vi "DCPower_RECONFIGURE_VoltageOrChannelname_AfterJSONfile_REFERENCE_byChannel.vi"(3 "error in":errorcluster, 4 "ColorPalette":T2=[16711686, 65351, 8978420, 14474240, 16139007, 16752640, 8958719, 16758973, 16777215, 46792, 11992992, 12961221, 16763690, 12600063, 16711835, 2953983, 40796, 13111296, 13352613, 9221011, 12964076, 12819897, 65442, 16776704, 14540253, 16740729, 10658047, 10813344, 16753521, 13413843, 8691115, 10339240, 14401205, 16746704, 7467519, 16775978, 13872558, 11387603, 13354405, 10420227, 13107364, 4060, 35208, 11817216, 7566080, 40796, 7539456, 2837073, 6372186, 7499083, 10648702, 16757152], 5 "VISAPowerInfoInputArray":T3[](array[typedef]), 6 "DCPowerInformationArrayOutput_byChannel_input":T1(array[cluster])) -> (0 "error out":errorcluster, 1 "VISAPowerInfoOutputArray":T3[](array[typedef]), 2 "DCPowerInformationArrayOutput_byChannel_output":T1(array[cluster]))   [LabVIEW 2019]
uses:
  Controls/PlotColorArray.ctl
  Controls/VISA_power_Control.ctl
panel:
  in  "Current Reset Value (A)":dbl
  out "Measured Voltage":dbl[](array[numeric])
  out "Measured Currents":dbl[](array[numeric])
  out "Configuration Echo":string
  out "Parameter Configuration Echo":string[][](array[string])
  in  "Channel Names":string[](array[string])
  in  "Change VISA Configurations":bool
  in  "Combination Scheme":u16(ring) items=["OFF", "SERIES", "PARALLEL"]
  in  "Which Channels to Parallelize":u16(ring) items=["I1+I2", "ALL", "I2+I3"]
  in  "Current Limit Channel 3":dbl
  in  "Current Limit Channel 2":dbl
  in  "Current Limit Channel 1":dbl
  in  "Voltage Channel 3":dbl
  in  "Voltage Channel 2":dbl
  in  "Voltage Channel 1":dbl
  in  "visa power channel select":u16(ring) items=["GPIB0::3::INSTR; channel names :channel1,channel2,channel3"]
  in  "Power On":bool
  in  "Change DC Power Channel Name":bool
  in  "Change DC Power Voltage":bool
  out "Current Measured (A)":dbl
  out "Voltage Measured (V)":dbl
  in  "Channel Name (str)":string
  in  "Voltage Level (V)":dbl
  out "Current Measured All (A)":dbl[][](array[numeric])
  out "Voltage Measured All (V)":dbl[][](array[numeric])
  out "Current Waveform Array":waveform(dbl)[](graph)
  out "Voltage Waveform Array":waveform(dbl)[](graph)
  in  "dc power channel select":u16(ring) items=["Slot_4_PXIe4139; channel number:  0; channel name: Red 5v", "Slot_5_PXIe4139; channel number:  0; channel name: Orange 3.3v_6780", "Slot_6_PXIe4139; channel number:  0; channel name: Yellow 1.8v", "PXIe4163; channel number:  0; channel name: Green 3.3v", "PXIe4163; channel number:  1; channel name: Blue 2.6v VATT"]
  in  "End Reconfig":bool
  # "Nothing to see behind here, surely"
  # "Change Parameters"
  # "MEASURED OUTPUTS (MAY NEED TO PRESS APPLY A FEW TIMES TO SEE ACTUAL OUTPUT)"
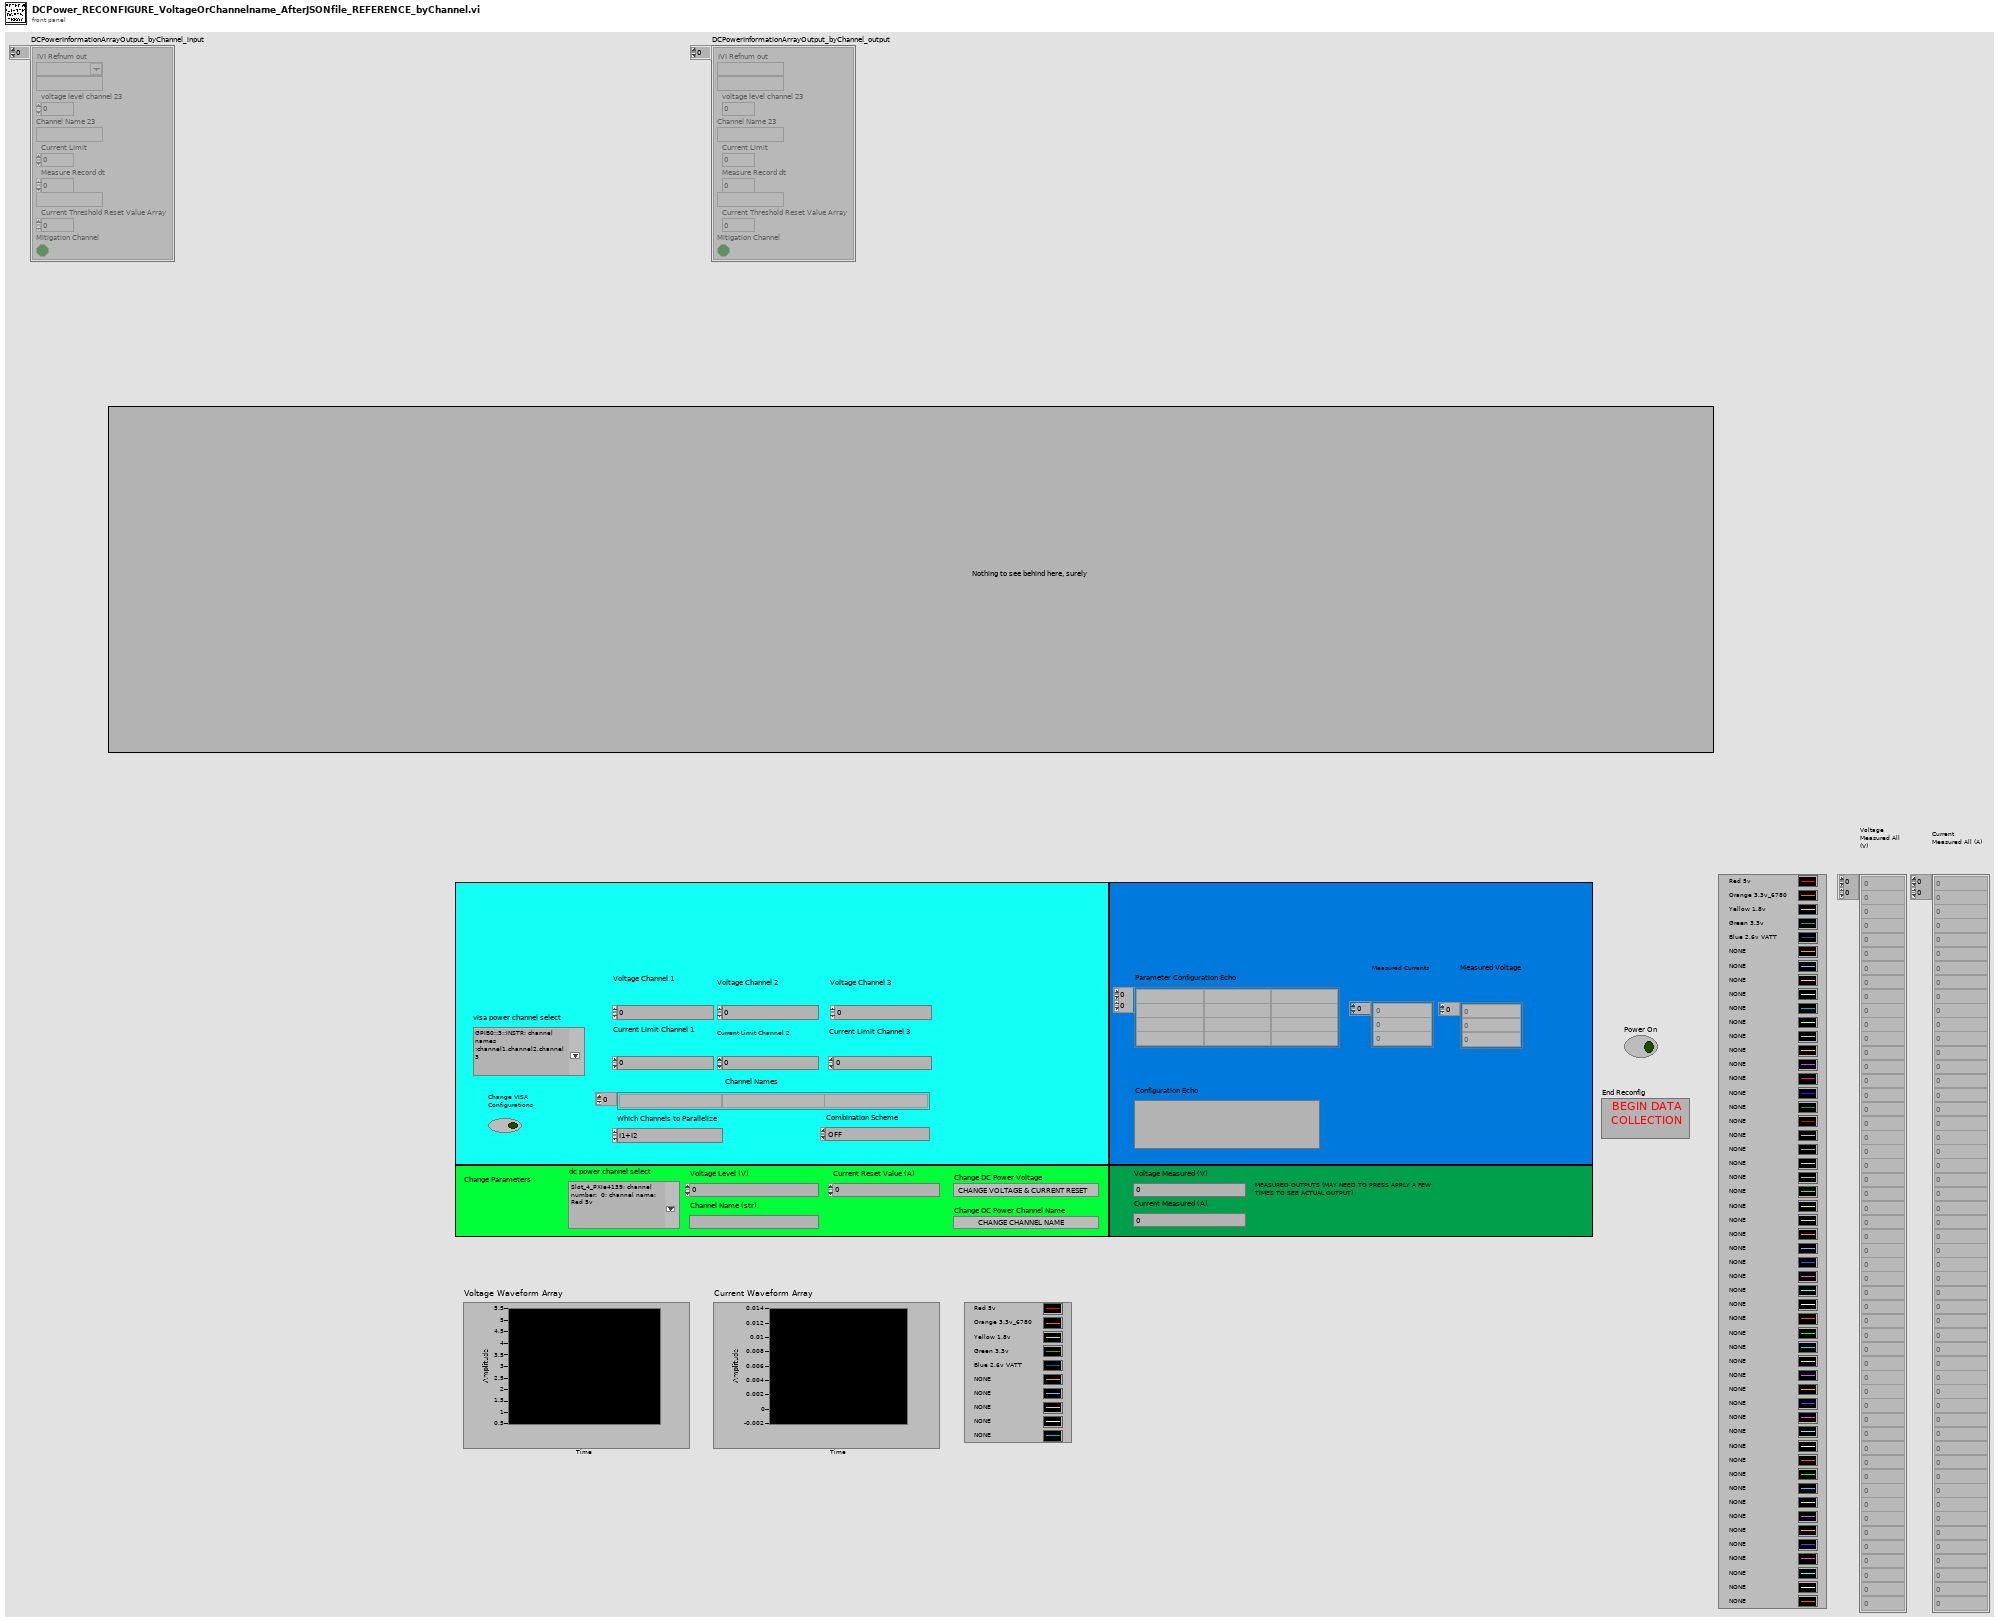
[diagram p1: front panel]
types:
  T1 = cluster{"IVI Refnum out":refnum<k15>, string, "voltage level channel 23":dbl, "Channel Name 23":string, "Current Limit":dbl, "Measure Record dt":dbl, string, "Current Threshold Reset Value Array":dbl, "Mitigation Channel":bool}[]
  T2 = typedef "PlotColorArray.ctl" = u32[]
  T3 = typedef "VISA_power_Control.ctl" = cluster{"VISA resource name":refnum<visa-resource-name>, "Active Channel List":string, "Active Channel Array":string[], "Input Array (Voltage,Current_Limit)":dbl[], "Input Array (Voltage,Current_Limit)":dbl[], "Channel Names":string[], "read buffer":string, "Channel Names Array":string[]}
  T4 = cluster{"IVI Refnum out":refnum<k15>, string, "voltage level channel 23":dbl, "Channel Name 23":string, "Current Limit":dbl, "Measure Record dt":dbl, string}[]
  T5 = typedef "LVStringsAndValuesArrayTypeDef_U16.ctl" = cluster{"String":string, "Value":u16}[]
  T6 = cluster{"VISA resource name":refnum<visa-resource-name>, "Active Channel List":string, "Active Channel Array":string[], "Input Array (Voltage,Current_Limit)":dbl[], "Input Array (Voltage,Current_Limit)":dbl[], "Channel Names":string[], "read buffer":string, "Channel Names":string[]}
  T7 = cluster{"IVI Refnum out":refnum<k15>, string, "voltage level channel 23":dbl, "Channel Name 23":string, "Current Limit":dbl, "Measure Record dt":dbl, string, "Current Threshold Reset Value Array":dbl, "Mitigation Channel":bool}
  T8 = cluster{"IVI Refnum out":refnum<k15>, string, "voltage level channel 23":dbl, "Channel Name (str)":string, "Current Limit":dbl, "Measure Record dt":dbl, string, "Current Threshold Reset Value Array":dbl, "Mitigation Channel":bool}
  T9 = cluster{"instrument handle out":refnum<k15>, string, "Voltage Level (V)":dbl, "Channel Name 23":string, "Current Limit":dbl, "Measure Record dt":dbl, string, "Current Reset Value (A)":dbl, "Mitigation Channel":bool}
  T10 = cluster{"IVI Refnum out":refnum<k15>, "String List":string, string[], dbl[], string[], dbl[], dbl[], string[], dbl[], bool[]}[]
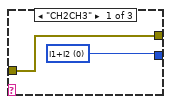
[diagram p4: hidden frame]
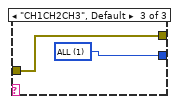
[diagram p5: hidden frame]
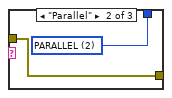
[diagram p6: hidden frame]
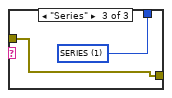
[diagram p7: hidden frame]
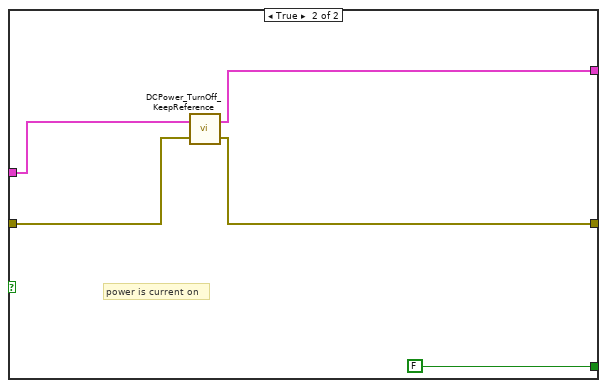
[diagram p9: hidden frame]
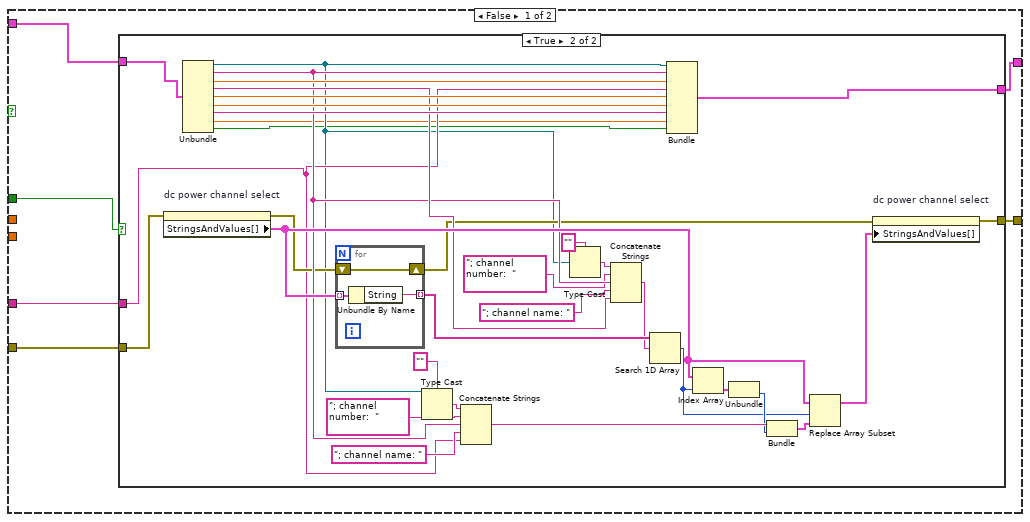
[diagram p10: hidden frame]
diagram:
  (unwired) T4 [] ("DCPowerInformation_byChannel_input")
  n1 = flat-sequence {
    tunnel: "DCPowerInformationArrayOutput_byChannel_input" -> [w16]
    tunnel: [w16] -> w12
    tunnel: [w15] -> w11
    tunnel: "error in" -> [w15]
    tunnel: [w13] -> w6
    tunnel: "VISAPowerInfoInputArray" -> [w13]
    tunnel: w12 -> [w34]
    tunnel: w11 -> [w47]
    tunnel: [w34] -> w10
    tunnel: [w17] -> w9
    tunnel: w6 -> [w28]
    tunnel: [w28] -> w5
    tunnel: w10 -> [w94]
    tunnel: w9 -> [w93]
    tunnel: [w92] -> w8
    tunnel: [w91] -> w1
    tunnel: w5 -> [w87]
    tunnel: [w86] -> w3
    frame #0 {
      n2 = local write "Power On"(FALSE ("Power On")) -> ()
    }
    frame #1 {
      n3 = Bundle("concatenated string"="pseudo", -1) -> (w46:cluster{"concatenated string":string, i32})  [unwired: 1 in]
      n4 = Build Array(w46) -> (w45:cluster{"concatenated string":string, i32}[])
      n5 = property on="dc power channel select" class="Ring (strict)"(error in=w47, "StringsAndValues[]"=w45) -> (error out=w48:errorcluster)  [unwired: 1 in, 1 out]
      n6 = property on="dc power channel select" class="Ring (strict)"(error in=w48) -> (error out=w49:errorcluster, "StringsAndValues[]"=w50:T5)  [unwired: 1 in, 1 out]
      n7 = for {
        tunnel: w34 -> [w76] mode=indexing
        shift-right: [w71] -> _
        shift-left: w50 -> [w73]
        shift-right: [w74] -> w42
        shift-left: w49 -> [w85]
        i -> [w75]
        n8 = Unbundle(w76) -> ("IVI Refnum out"=w84:refnum<k15>, w80:string, "Channel Name 23"=w78:string)  [unwired: 6 out]
        n9 = Type Cast(type="", x=w84) -> (*(type *) &x=w82:string)
        n10 = Concatenate Strings(w82, "; channel number:  " ("string"), w80, "; channel name: " ("string"), w78) -> (w77:string)
        n11 = Bundle(w77, w75) -> (w72:cluster{string, i32})  [unwired: 1 in]
        n12 = Build Array (concatenate)(w73, w72) -> (w71:cluster{"String":string, "Value":i32}[])
        n13 = property on="dc power channel select" class="Ring (strict)"(error in=w85, "StringsAndValues[]"=w71) -> (error out=w74:errorcluster)  [unwired: 1 in, 1 out]
      }
      n14 = property on="dc power channel select" class="Ring (strict)"(error in=w42) -> (error out=w41:errorcluster, "StringsAndValues[]"=w37:T5)  [unwired: 1 in, 1 out]
      n15 = for {
        tunnel: w37 -> [w70] mode=indexing
        shift-right: [w68] -> _
        shift-left: w41 -> [w68]
        tunnel: [w69] -> w39 mode=indexing
        n16 = Unbundle By Name(w70) -> ("Value"=w69:u16)
      }
      n17 = Search 1D Array(1D array=w39, element=u16 65535) -> (index of element=w40:i32)  [unwired: 1 in]
      n18 = Delete From Array(array=w37, index=w40) -> (array with subset deleted=w36:T5)  [unwired: 1 in, 1 out]
      n19 = property on="dc power channel select" class="Ring (strict)"(error in=w41, "StringsAndValues[]"=w36) -> (error out=w35:errorcluster)  [unwired: 1 in, 1 out]
      n20 = property on="dc power channel select" class="Ring (strict)" props=["StringsAndValues[]"](error in=w35) -> (error out=w29:errorcluster)  [unwired: 1 in, 2 out]
      n21 = Bundle("concatenated string"="pseudo", -1) -> (w31:cluster{"concatenated string":string, i32})  [unwired: 1 in]
      n22 = Build Array(w31) -> (w30:cluster{"concatenated string":string, i32}[])
      n23 = property on="visa power channel select" class="Ring (strict)"(error in=w29, "StringsAndValues[]"=w30) -> (error out=w27:errorcluster)  [unwired: 1 in, 1 out]
      n24 = property on="visa power channel select" class="Ring (strict)"(error in=w27) -> (error out=w26:errorcluster, "StringsAndValues[]"=w25:T5)  [unwired: 1 in, 1 out]
      n25 = for {
        shift-right: [w56] -> w24
        shift-left: w26 -> [w57]
        shift-right: [w55] -> _
        shift-left: w25 -> [w58]
        tunnel: w28 -> [w67] mode=indexing
        i -> [w60]
        n26 = Unbundle(w67) -> ("VISA resource name"=w66:refnum<visa-resource-name>, "Channel Names Array"=w54:string[])  [unwired: 6 out]
        n27 = call "StringArray2StringList.vi"("String Array"=w54) -> ("String List"=w62:string)
        n28 = Type Cast(type="", x=w66) -> (*(type *) &x=w64:string)
        n29 = Concatenate Strings(w64, "; channel names :" ("string"), w62) -> (w61:string)
        n30 = Bundle(w61, w60) -> (w59:cluster{string, i32})  [unwired: 1 in]
        n31 = Build Array (concatenate)(w58, w59) -> (w55:cluster{"String":string, "Value":i32}[])
        n32 = property on="visa power channel select" class="Ring (strict)"(error in=w57, "StringsAndValues[]"=w55) -> (error out=w56:errorcluster)  [unwired: 1 in, 1 out]
      }
      n33 = property on="visa power channel select" class="Ring (strict)"(error in=w24) -> (error out=w18:errorcluster, "StringsAndValues[]"=w20:T5)  [unwired: 1 in, 1 out]
      n34 = for {
        tunnel: w20 -> [w53] mode=indexing
        shift-right: [w51] -> _
        shift-left: w20 -> [w51]
        tunnel: [w52] -> w22 mode=indexing
        n35 = Unbundle By Name(w53) -> ("Value"=w52:u16)
      }
      n36 = Search 1D Array(1D array=w22, element=u16 65535) -> (index of element=w23:i32)  [unwired: 1 in]
      n37 = Delete From Array(array=w20, index=w23) -> (array with subset deleted=w19:T5)  [unwired: 1 in, 1 out]
      n38 = property on="visa power channel select" class="Ring (strict)"(error in=w18, "StringsAndValues[]"=w19) -> (error out=w17:errorcluster)  [unwired: 1 in, 1 out]
    }
    frame #2 {
      n39 = while {
        shift-right: [w95] -> w91
        shift-left: w94 -> [w138]
        shift-right: [w118] -> w92
        shift-left: w93 -> [w114]
        tunnel: "ColorPalette" -> [w136]
        shift-right: [w124] -> _
        shift-left: FALSE (".not. x?") -> [w102]
        shift-right: [w109] -> _
        shift-left: u16 0 -> [w106]
        shift-right: [w98] -> w86
        shift-left: w87 -> [w110]
        i -> [w105]
        stop <- w137 stop-if-true
        # "Need to add channel number cofiguration(position eventually)"
        n40 = property on="visa power channel select" class="Ring (strict)"(error in=w114) -> (error out=w113:errorcluster, "StringsAndValues[]"=w116:T5)  [unwired: 1 in, 1 out]
        n41 = Index Array(array=w116, index="visa power channel select") -> (element=w115:cluster{"String":string, "Value":u16})
        n42 = Unbundle(w115) -> ("Value"=w109:u16)  [unwired: 1 out]
        n43 = Not Equal?(x=w109, y=w106) -> (x != y?=w108:bool)
        n44 = Equal To 0?(x=w105) -> (x = 0?=w107:bool)
        n45 = Or(x=w108, y=w107) -> (x .or. y?=w104:bool)
        n46 = case shown="True" w104 {
          tunnel: w110 -> [_ w232]
          tunnel: w109 -> [_ w233]
          tunnel: [w197 w208] -> w112
          tunnel: w113 -> [w197 w211]
          frame False {
          }
          frame True {
            n47 = Index Array(array=w232, index=w233) -> (element=w231:T3)
            n48 = Unbundle(w231) -> ("Input Array (Voltage,Current_Limit)"=w221:dbl[], "Input Array (Voltage,Current_Limit)"=w220:dbl[], "Channel Names"=w207:string[], "read buffer"=w206:string)  [unwired: 4 out]
            n49 = Index Array(array=w221, index=0) -> (element=w225:dbl)
            n50 = call <vilib>:"Space Constant.vi"() -> ("String"=w205:string)
            n51 = property on="Voltage Channel 1" class="DigNum (strict)"(error in=w211, "Value"=w225) -> (error out=w230:errorcluster)  [unwired: 1 in, 1 out]
            n52 = Index Array(array=w221, index=1) -> (element=w224:dbl)
            n53 = Match Pattern(string=w206, regular expression=w205) -> (before substring=w204:string, after substring=w201:string)  [unwired: 1 in, 2 out]
            n54 = property on="Voltage Channel 2" class="DigNum (strict)"(error in=w230, "Value"=w224) -> (error out=w229:errorcluster)  [unwired: 1 in, 1 out]
            n55 = Index Array(array=w221, index=2) -> (element=w223:dbl)
            n56 = property on="Voltage Channel 3" class="DigNum (strict)"(error in=w229, "Value"=w223) -> (error out=w228:errorcluster)  [unwired: 1 in, 1 out]
            n57 = Index Array(array=w220, index=0) -> (element=w222:dbl)
            n58 = property on="Current Limit Channel 1" class="DigNum (strict)"(error in=w228, "Value"=w222) -> (error out=w226:errorcluster)  [unwired: 1 in, 1 out]
            n59 = Index Array(array=w220, index=1) -> (element=w219:dbl)
            n60 = property on="Current Limit Channel 2" class="DigNum (strict)"(error in=w226, "Value"=w219) -> (error out=w227:errorcluster)  [unwired: 1 in, 1 out]
            n61 = Index Array(array=w220, index=2) -> (element=w218:dbl)
            n62 = property on="Current Limit Channel 3" class="DigNum (strict)"(error in=w227, "Value"=w218) -> (error out=w203:errorcluster)  [unwired: 1 in, 1 out]
            n63 = case shown="\"NONE\", Default" w204 {
              tunnel: w203 -> [w240 w242 w244]
              tunnel: [w241 w243 w245] -> w202
              tunnel: [w240 w242 w244] -> w199
              frame "NONE", Default {
                w241 = u16 0 items=["OFF", "SERIES", "PARALLEL"] ("Combination Scheme")
              }
              frame "Parallel" {
                w243 = u16 2 items=["OFF", "SERIES", "PARALLEL"] ("Combination Scheme")
              }
              frame "Series" {
                w245 = u16 1 items=["OFF", "SERIES", "PARALLEL"] ("Combination Scheme")
              }
            }
            n64 = case shown="\"CH1CH2\"" w201 {
              tunnel: [w235 w237 w239] -> w200
              tunnel: [w234 w236 w238] -> w198
              tunnel: w199 -> [w234 w236 w238]
              frame "CH2CH3" {
                w235 = u16 0 items=["I1+I2", "ALL", "I2+I3"] ("Which Channels to Parallelize")
              }
              frame "CH1CH2" {
                w237 = u16 0 items=["I1+I2", "ALL", "I2+I3"] ("Which Channels to Parallelize")
              }
              frame "CH1CH2CH3", Default {
                w239 = u16 1 items=["I1+I2", "ALL", "I2+I3"] ("Which Channels to Parallelize")
              }
            }
            n65 = property on="Combination Scheme" class="Ring (strict)"(error in=w198, "Value"=w202) -> (error out=w210:errorcluster)  [unwired: 1 in, 1 out]
            n66 = property on="Which Channels to Parallelize" class="Ring (strict)"(error in=w210, "Value"=w200) -> (error out=w209:errorcluster)  [unwired: 1 in, 1 out]
            n67 = property on="Channel Names" class="Arr (strict)"(error in=w209, "Value"=w207) -> (error out=w208:errorcluster)  [unwired: 1 in, 1 out]
          }
        }
        n68 = Exclusive Or(1:"Power On", 2:w102) -> (0:w101:bool)
        n69 = Or(x="Change VISA Configurations", y=w101) -> (x .or. y?=w99:bool)
        n70 = case shown="True" w99 {
          tunnel: w112 -> [w140 w170]
          tunnel: [w140 w143] -> w111
          tunnel: w110 -> [w139 w156]
          tunnel: w109 -> [_ w169]
          tunnel: [w139 w142] -> w98
          tunnel: "Power On" -> [_ w151]
          tunnel: "visa power channel select" -> [_ w146]
          frame False {
          }
          frame True {
            n71 = Index Array(array=w156, index=w169) -> (element=w155:T3)
            n72 = Unbundle By Name(w155) -> ("VISA resource name"=w154:refnum<visa-resource-name>)
            n73 = Build Array("Current Limit Channel 1", "Current Limit Channel 2", "Current Limit Channel 3") -> (w161:dbl[])
            n74 = Build Array("Voltage Channel 1", "Voltage Channel 2", "Voltage Channel 3") -> (w162:dbl[])
            n75 = Build Array(w162, w161) -> (w160:dbl[][])
            n76 = Transpose 2D Array(2D array=w160) -> (transposed array=w159:dbl[][])
            n77 = call "VISA_Keithley2230G_ConfigureInstrument_V1.vi"("VISA resource name"=w154, "VISAPowerInfoInputArray"=w156, "Input Array (Voltage,Current_Limit)"=w159, "Combination Scheme"="Combination Scheme", "Which Channels to Parallelize"="Which Channels to Parallelize", "error in"=w170, "POWER STATUS IN"=w151, "Channel Names"="Channel Names", "json configured?"=TRUE) -> ("VISAPowerInfoOutputArray"=w148:T3[], "Configuration Echo"=→"Configuration Echo":string, "Parameter Configuration Echo"=→"Parameter Configuration Echo":string[][], "error out"=w149:errorcluster)  [unwired: 6 in, 1 out]
            n78 = flat-sequence {
              tunnel: w149 -> [w192]
              tunnel: w148 -> [w172]
              tunnel: "Channel Names" -> [w179]
              tunnel: w146 -> [w171]
              tunnel: [w176] -> w145
              tunnel: [w175] -> w144
              tunnel: [w173] -> w141
              tunnel: w145 -> [w196]
              tunnel: w144 -> [w195]
              tunnel: [w194] -> w143
              tunnel: [w193] -> w142
              tunnel: w141 -> [w193]
              frame #0 {
                n79 = property on="visa power channel select" class="Ring (strict)"(error in=w192) -> (error out=w176:errorcluster, "StringsAndValues[]"=w177:T5)  [unwired: 1 in, 1 out]
                n80 = Index Array(array=w172, index=w171) -> (element=w191:T3)
                n81 = Unbundle(w191) -> ("VISA resource name"=w180:refnum<visa-resource-name>, "Active Channel List"=w190:string, "Active Channel Array"=w186:string[], "Input Array (Voltage,Current_Limit)"=w187:dbl[], "Input Array (Voltage,Current_Limit)"=w188:dbl[], "read buffer"=w189:string)  [unwired: 2 out]
                n82 = Bundle("VISA resource name"=w180, "Active Channel List"=w190, "Active Channel Array"=w186, "Input Array (Voltage,Current_Limit)"=w187, "Input Array (Voltage,Current_Limit)"=w188, "Channel Names"=w179, "read buffer"=w189, "Channel Names"=w179) -> (w174:T6)  [unwired: 1 in]
                n83 = call "StringArray2StringList.vi"("String Array"=w179) -> ("String List"=w182:string)
                n84 = Type Cast(type="", x=w180) -> (*(type *) &x=w184:string)
                n85 = Concatenate Strings(w184, "; channel names :" ("string"), w182) -> (w181:string)
                n86 = Replace Array Subset(array=w172, new element=w174, index=w171) -> (w173:T3[])
                n87 = Bundle(w181, "visa power channel select"=w171) -> (w178:cluster{string, "visa power channel select":u16})  [unwired: 1 in]
                n88 = Replace Array Subset(array=w177, new element=w178) -> (w175:T5)  [unwired: 1 in]
              }
              frame #1 {
                n89 = property on="visa power channel select" class="Ring (strict)"(error in=w196, "StringsAndValues[]"=w195) -> (error out=w194:errorcluster)  [unwired: 1 in, 1 out]
              }
            }
          }
        }
        n90 = Index Array(array=w138, index="dc power channel select") -> (element=w130:T7)
        n91 = case shown="True" "Change DC Power Voltage" {
          tunnel: w130 -> [w269 w315]
          tunnel: [w266 w312] -> w131
          tunnel: [w267 w313] -> w135
          tunnel: w111 -> [w270 w314]
          tunnel: "Channel Name (str)" -> [w268 _]
          tunnel: "Voltage Level (V)" -> [_ w311]
          tunnel: "Change DC Power Channel Name" -> [w265 _]
          tunnel: "Current Reset Value (A)" -> [_ w310]
          frame False {
            n92 = case shown="True" w265 {
              tunnel: w270 -> [w272 w280]
              tunnel: w269 -> [w271 w279]
              tunnel: w268 -> [_ w278]
              tunnel: [w272 w276] -> w267
              tunnel: [w271 w275] -> w266
              frame False {
              }
              frame True {
                n93 = property on="dc power channel select" class="Ring (strict)"(error in=w280) -> (error out=w288:errorcluster, "StringsAndValues[]"=w294:T5)  [unwired: 1 in, 1 out]
                n94 = Unbundle(w279) -> ("IVI Refnum out"=w277:refnum<k15>, w289:string, "voltage level channel 23"=w304:dbl, "Channel Name 23"=w291:string, "Current Limit"=w303:dbl, "Measure Record dt"=w302:dbl, w305:string, "Current Threshold Reset Value Array"=w274:dbl, "Mitigation Channel"=w273:bool)
                n95 = for {
                  tunnel: w294 -> [w308] mode=indexing
                  shift-right: [w306] -> w287
                  shift-left: w288 -> [w306]
                  tunnel: [w307] -> w301 mode=indexing
                  n96 = Unbundle By Name(w308) -> ("String"=w307:string)
                }
                n97 = Type Cast(type="", x=w277) -> (*(type *) &x=w299:string)
                n98 = Concatenate Strings(w299, "; channel number:  " ("string"), w289, "; channel name: " ("string"), w278) -> (w300:string)
                n99 = Type Cast(type="", x=w277) -> (*(type *) &x=w292:string)
                n100 = Concatenate Strings(w292, "; channel number:  " ("string"), w289, "; channel name: " ("string"), w291) -> (w290:string)
                n101 = Search 1D Array(1D array=w301, element=w290) -> (index of element=w295:i32)  [unwired: 1 in]
                n102 = Bundle("IVI Refnum out"=w277, w289, "voltage level channel 23"=w304, "Channel Name (str)"=w278, "Current Limit"=w303, "Measure Record dt"=w302, w305, "Current Threshold Reset Value Array"=w274, "Mitigation Channel"=w273) -> (w275:T8)  [unwired: 1 in]
                n103 = Index Array(array=w294, index=w295) -> (element=w298:cluster{"String":string, "Value":u16})
                n104 = Unbundle(w298) -> ("Value"=w297:u16)  [unwired: 1 out]
                n105 = Bundle(w300, "Value"=w297) -> (w296:cluster{string, "Value":u16})  [unwired: 1 in]
                n106 = Replace Array Subset(array=w294, new element=w296, index=w295) -> (w293:T5)
                n107 = property on="dc power channel select" class="Ring (strict)"(error in=w287, "StringsAndValues[]"=w293) -> (error out=w276:errorcluster)  [unwired: 1 in, 1 out]
              }
            }
          }
          frame True {
            n108 = Unbundle(w315) -> ("IVI Refnum out"=w320:refnum<k15>, w316:string, "Channel Name 23"=w321:string, "Current Limit"=w323:dbl, "Measure Record dt"=w322:dbl, w324:string, "Mitigation Channel"=w309:bool)  [unwired: 2 out]
            n109 = call <instrlib>:"niDCPower Configure Voltage Level.vi"("error in (no error)"=w314, "voltage level"=w311, "channel name"=w316, "instrument handle"=w320) -> ("error out"=w319:errorcluster, "instrument handle out"=w318:refnum<k15>)  [unwired: 6 in]
            n110 = call <instrlib>:"niDCPower Commit With Channels.vi"("error in (no error)"=w319, "channel name"=w316, "instrument handle"=w318) -> ("error out"=w313:errorcluster, "instrument handle out"=w317:refnum<k15>)  [unwired: 7 in]
            n111 = Bundle("instrument handle out"=w317, w316, "Voltage Level (V)"=w311, "Channel Name 23"=w321, "Current Limit"=w323, "Measure Record dt"=w322, w324, "Current Reset Value (A)"=w310, "Mitigation Channel"=w309) -> (w312:T9)  [unwired: 1 in]
          }
        }
        n112 = Exclusive Or(1:"Power On", 2:w102) -> (0:w123:bool)
        n113 = Replace Array Subset(array=w138, new element=w131, index="dc power channel select") -> (w95:T1)
        n114 = call "Convert_ChannelReferenceArray_2_InstrumentReferenceArray.vi"("error in"=w135, "DCPowerInformation_byChannel_input"=w95) -> ("error out"=w127:errorcluster, "DCPower_byInstrument_output"=w122:T10)
        n115 = Or(x="Change DC Power Channel Name", y="Change DC Power Voltage") -> (x .or. y?=w119:bool)
        n116 = case shown="True" w123 {
          tunnel: w127 -> [w247 w254]
          tunnel: [w247 w253] -> w126
          tunnel: w122 -> [w248 w249]
          tunnel: [w248 w252] -> w125
          tunnel: w102 -> [w246 w251]
          tunnel: [w246 w250] -> w124
          frame False {
            # "power button has not been toggled"
          }
          frame True {
            # "power button has been toggled"
            n117 = case shown="False" w251 {
              tunnel: w254 -> [w259 w264]
              tunnel: [w256 w262] -> w253
              tunnel: [w257 w263] -> w252
              tunnel: [TRUE (".not. x?") FALSE (".not. x?")] -> w250
              tunnel: w249 -> [w258 w260]
              frame False {
                # "power is currently off. Turning on"
                n118 = call "DCPower_Reconfig_byInstrument_perChannel.vi"("error in (no error)"=w259, "DCPower_byInstrument_input"=w258) -> ("error out"=w256:errorcluster, "DCPowerInformation_byInstrument"=w257:T10)
              }
              frame True {
                # "power is current on"
                n119 = call "DCPower_TurnOff_KeepReference.vi"("error in (no error)"=w264, "DCPower_byInstrument_input"=w260) -> ("error out"=w262:errorcluster, "DCPower_byInstrument_output"=w263:T10)
              }
            }
          }
        }
        n120 = case shown="True" "Power On" {
          tunnel: w125 -> [w325 w336]
          tunnel: w126 -> [w326 w330]
          tunnel: [w326 w339] -> w133
          tunnel: w136 -> [_ w338]
          tunnel: [w325 w337] -> _
          tunnel: "dc power channel select" -> [_ w333]
          tunnel: w119 -> [_ w332]
          tunnel: w98 -> [_ w331]
          frame False {
          }
          frame True {
            # "Fetching some data to confirm part is powered on properly. Indicators are shown to the right"
            # "Making all the colors and names of the chart \"none\" so empty names are called \"none\""
            # "renaming the legend and the colors of the chart"
            # "closing the instrument if it is not configured anymore\nthis should never trigger"
            n121 = for {
              tunnel: w331 -> [w363] mode=indexing
              shift-right: [w360] -> w328
              shift-left: w330 -> [w361]
              tunnel: [w359] -> w327 mode=concatenating
              tunnel: [w358] -> w329 mode=concatenating
              w366 = u32 20 ("byte count")
              n122 = Unbundle By Name(w363) -> ("VISA resource name"=w362:refnum<visa-resource-name>)
              n123 = VISA Open(error in (no error)=w361, VISA resource name=w362) -> (VISA resource name=w369:refnum<visa-resource-name>, error out=w368:errorcluster)  [unwired: 3 in]
              n124 = VISA Write(VISA resource name=w369, write buffer="FETC:CURR? ALL", error in (no error)=w368) -> (VISA resource name out=w370:refnum<visa-resource-name>, error out=w367:errorcluster)  [unwired: 1 out]
              n125 = VISA Read(VISA resource name=w370, byte count=w366, error in (no error)=w367) -> (VISA resource name out=w375:refnum<visa-resource-name>, read buffer=w357:string, error out=w376:errorcluster)  [unwired: 1 out]
              n126 = call "StringList2StringArray.vi"("Active Channel Numbers String"=w357) -> ("Array"=w356:string[])
              n127 = VISA Write(VISA resource name=w375, write buffer="FETC:VOLT? ALL", error in (no error)=w376) -> (VISA resource name out=w374:refnum<visa-resource-name>, error out=w371:errorcluster)  [unwired: 1 out]
              n128 = VISA Read(VISA resource name=w374, byte count=w366, error in (no error)=w371) -> (VISA resource name out=w373:refnum<visa-resource-name>, read buffer=w355:string, error out=w372:errorcluster)  [unwired: 1 out]
              n129 = Fract/Exp String To Number(string=w356) -> (number=w359:dbl[])  [unwired: 3 in, 1 out]
              n130 = call "StringList2StringArray.vi"("Active Channel Numbers String"=w355) -> ("Array"=w354:string[])
              n131 = VISA Close(VISA resource name=w373, error in (no error)=w372) -> (error out=w360:errorcluster)
              n132 = Fract/Exp String To Number(string=w354) -> (number=w358:dbl[])  [unwired: 3 in, 1 out]
            }
            "Measured Currents" <- w327
            "Measured Voltage" <- w329
            n133 = for {
              tunnel: [w435] -> w337 mode=indexing if=w424
              tunnel: w336 -> [w435] mode=indexing
              shift-right: [w426] -> w343
              shift-left: w328 -> [w433]
              n134 = Unbundle(w435) -> ("IVI Refnum out"=w434:refnum<k15>, "String List"=w429:string, w422:string[])  [unwired: 7 out]
              n135 = Equal?(x=w429, y="") -> (x = y?=w425:bool)
              n136 = call "StringArray2StringList.vi"("String Array"=w422) -> ("String List"=w428:string)
              n137 = call <instrlib>:"niDCPower Initiate With Channels.vi"("error in (no error)"=w433, "channel name"=w428, "instrument handle"=w434) -> ("error out"=w432:errorcluster, "instrument handle out"=w431:refnum<k15>)  [unwired: 7 in]
              n138 = call <instrlib>:"niDCPower Abort With Channels.vi"("error in (no error)"=w432, "channel name"=w428, "instrument handle"=w431) -> ("error out"=w427:errorcluster, "instrument handle out"=w423:refnum<k15>)  [unwired: 7 in]
              n139 = case shown="True" w425 {
                tunnel: w427 -> [w436 w439]
                tunnel: [w436 w437] -> w426
                tunnel: w423 -> [_ w438]
                frame False {
                }
                frame True {
                  n140 = call <instrlib>:"niDCPower Close.vi"("error in (no error)"=w439, "instrument handle"=w438) -> ("error out"=w437:errorcluster)  [unwired: 9 in]
                }
              }
              n141 = Not(x=w425) -> (.not. x?=w424:bool)
            }
            n142 = for {
              tunnel: w337 -> [w421] mode=indexing
              shift-right: [w418] -> w342
              shift-left: w343 -> [w417]
              n143 = Unbundle By Name(w421) -> ("IVI Refnum out"=w419:refnum<k15>, "String List"=w420:string)
              n144 = call <instrlib>:"niDCPower Initiate With Channels.vi"("error in (no error)"=w417, "channel name"=w420, "instrument handle"=w419) -> ("error out"=w418:errorcluster)  [unwired: 7 in, 1 out]
            }
            n145 = call "Convert_InstrumentReferenceArray_2_ChannelReferenceArray.vi"("error in (no error)"=w342, "DCPowerInformationClusterArray_Input"=w337) -> ("error out"=w345:errorcluster, "DCPowerInformationArrayOutput_byChannel"=w346:T1)
            n146 = for {
              shift-right: [w410] -> w344
              shift-left: w345 -> [w408]
              tunnel: w338 -> [_] mode=indexing
              i -> [w407]
              w406 = "NONE" ("Plot.Plot Name")
              n147 = property on="Current Waveform Array" class="WFChart (strict)"(error in=w408, "Active Plot"=w407, "Plot.Plot Name"=w406) -> (error out=w409:errorcluster)  [unwired: 1 in, 1 out]
              n148 = property on="Voltage Waveform Array" class="WFChart (strict)"(error in=w409, "Active Plot"=w407, "Plot.Plot Name"=w406) -> (error out=w410:errorcluster)  [unwired: 1 in, 1 out]
            }
            n149 = case shown="No Error" w344 {
              selector: w344 -> [w404 _]
              tunnel: [w404 w405] -> w348
              tunnel: w345 -> [_ w405]
              frame No Error {
              }
              frame Error {
              }
            }
            n150 = for {
              shift-right: [w401] -> w349
              shift-left: w348 -> [w402]
              tunnel: w346 -> [w400] mode=indexing
              tunnel: w338 -> [w399] mode=indexing
              tunnel: w338 -> [w398] mode=indexing
              i -> [w397]
              n151 = Unbundle By Name(w400) -> ("Channel Name 23"=w396:string)
              n152 = property on="Current Waveform Array" class="WFChart (strict)"(error in=w402, "Active Plot"=w397, "Plot.Plot Name"=w396, "Plot.Plot Color"=w399) -> (error out=w403:errorcluster)  [unwired: 1 in, 1 out]
              n153 = property on="Voltage Waveform Array" class="WFChart (strict)"(error in=w403, "Active Plot"=w397, "Plot.Plot Name"=w396, "Plot.Plot Color"=w398) -> (error out=w401:errorcluster)  [unwired: 1 in, 1 out]
            }
            n154 = case shown="Error .." w349 {
              selector: w349 -> [w389 _]
              tunnel: [w389 w390] -> w347
              tunnel: w348 -> [_ w390]
              frame No Error {
              }
              frame Error {
              }
            }
            n155 = for {
              N: 1000 -> [_]
              tunnel: w346 -> [w416]
              tunnel: timestamp(0 s since 1904-01-01) ("Initial Time") -> [w415]
              shift-right: [w413] -> w352
              shift-left: w347 -> [w414]
              tunnel: [w412] -> w350
              tunnel: [w411] -> w353
              n156 = call "Fetch&Process_Measurements_V4.vi"("DCPowerInformationArrayOutput_byChannel"=w416, "Initial Time"=w415, "error in (no error)"=w414) -> ("Current Waveform Array"=w411:waveform(dbl)[], "Voltage Waveform Array"=w412:waveform(dbl)[], "error out"=w413:errorcluster)  [unwired: 4 in, 6 out]
              "Current Waveform Array" <- w411
              "Voltage Waveform Array" <- w412
            }
            n157 = for {
              tunnel: w350 -> [w388] mode=indexing
              shift-right: [w387] -> w351
              shift-left: w352 -> [w387]
              tunnel: w353 -> [w386] mode=indexing
              tunnel: [w385] -> w334 mode=indexing
              tunnel: [w384] -> w335 mode=indexing
              n158 = Unbundle By Name(w386) -> ("Y"=w384:dbl[])
              n159 = Unbundle By Name(w388) -> ("Y"=w385:dbl[])
            }
            n160 = for {
              tunnel: w337 -> [w395] mode=indexing
              shift-right: [w391] -> w339
              shift-left: w351 -> [w392]
              n161 = Unbundle By Name(w395) -> ("IVI Refnum out"=w394:refnum<k15>, "String List"=w393:string)
              n162 = call <instrlib>:"niDCPower Abort With Channels.vi"("error in (no error)"=w392, "channel name"=w393, "instrument handle"=w394) -> ("error out"=w391:errorcluster)  [unwired: 7 in, 1 out]
            }
            n163 = case shown="True" w332 {
              tunnel: w335 -> [_ w383]
              tunnel: w334 -> [_ w382]
              tunnel: w333 -> [_ w379]
              frame False {
              }
              frame True {
                n164 = Index Array(array=w382, index (row)=w379, index (col)=0 ("disabled index (col)")) -> (element=→"Voltage Measured (V)":dbl)
                n165 = Index Array(array=w383, index (row)=w379, index (col)=0 ("disabled index (col)")) -> (element=→"Current Measured (A)":dbl)
                "Voltage Measured All (V)" <- w382
                "Current Measured All (A)" <- w383
              }
            }
          }
        }
        n166 = call "Time Delay2"("error in (no error)"=w133, "Delay Time (s)"=0.1) -> ("error out"=w118:errorcluster)  [unwired: 9 in]
        n167 = Or(x=w118, y="End Reconfig") -> (x .or. y?=w137:bool)
      }
    }
  }
  "error out" <- w8
  "VISAPowerInfoOutputArray" <- w3
  "DCPowerInformationArrayOutput_byChannel_output" <- w1
